vi "Scripting_ConnecorPaneRewiring.vi"(0 "ViRef":refnum<vi>, 1 "SubViThatHasChangedConnectorPane":path, 2 "OldConnectorPaneIndex":u32[](array[numeric]), 3 "NewConnectorPaneIndex":u32[](array[numeric]), 5 "error in (no error)":errorcluster) -> (19 "error out":errorcluster)   [LabVIEW 2020]
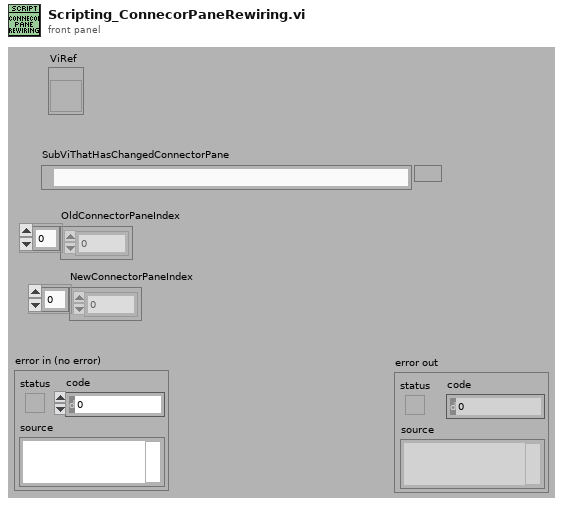
[diagram p1: front panel]
types:
  T1 = cluster{"New":refnum<vi>[], "Terminals[]":cluster{"Terminals[]":refnum<vi>[]}[]}
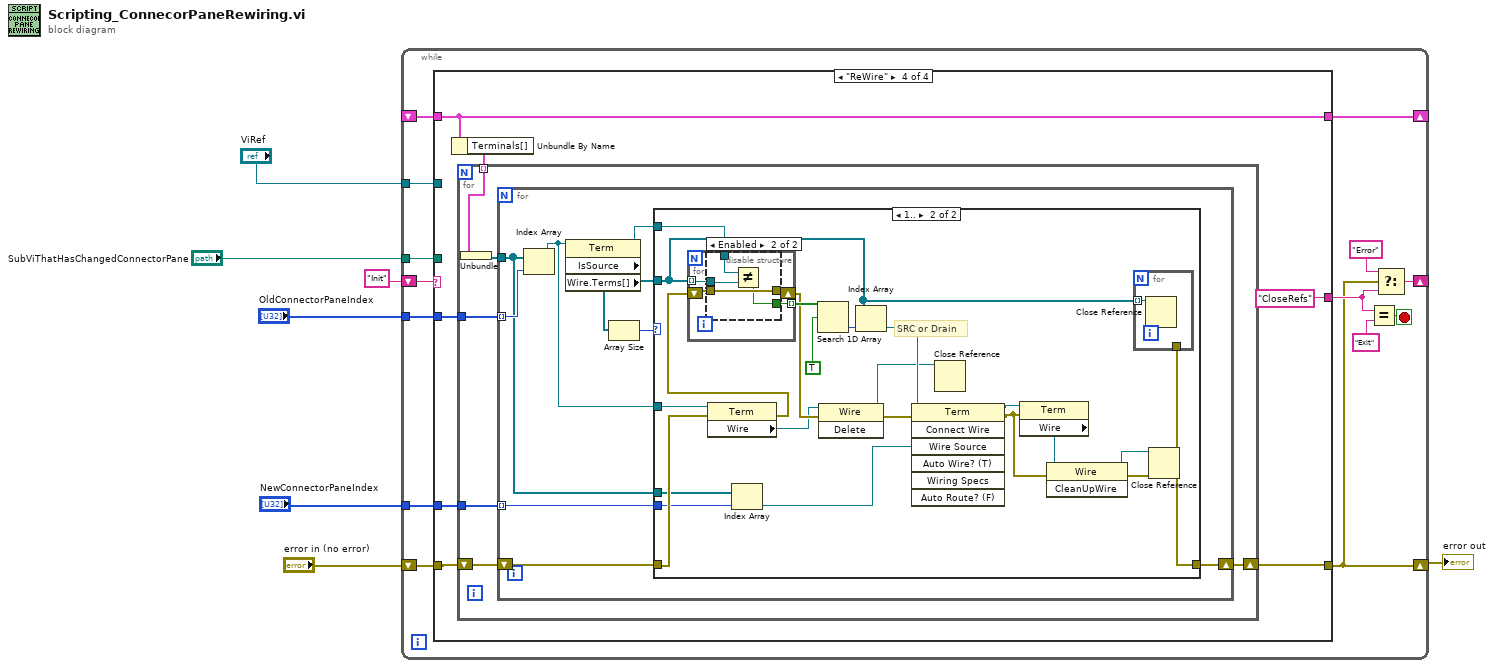
[diagram p0: block diagram]
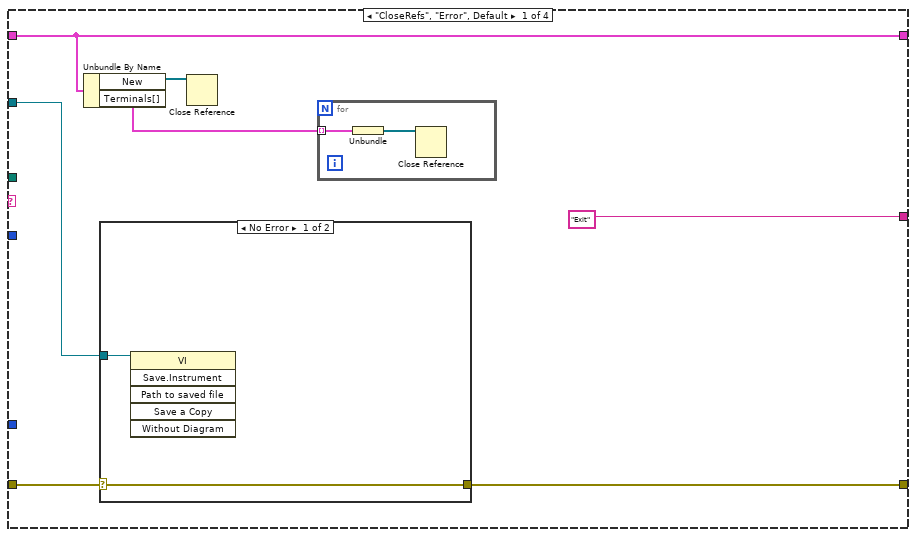
[diagram p2: hidden frame]
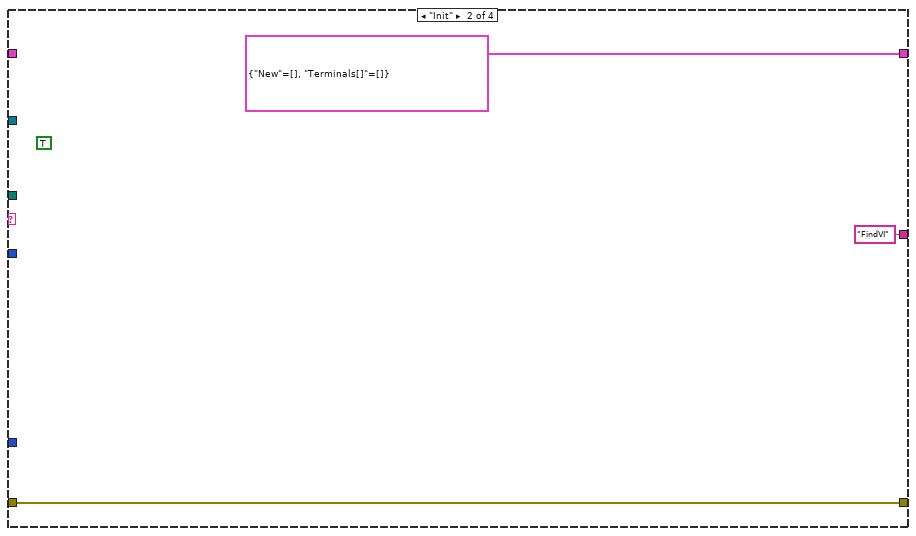
[diagram p4: hidden frame]
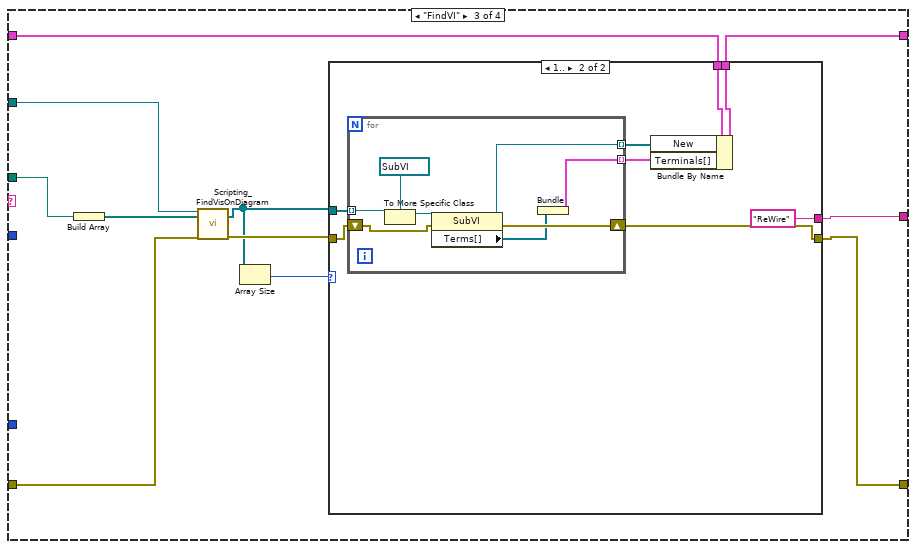
[diagram p5: hidden frame]
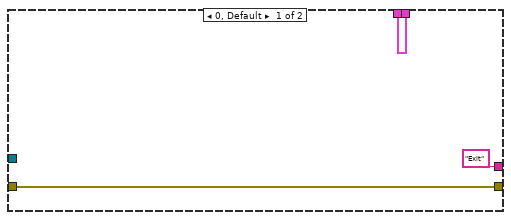
[diagram p6: hidden frame]
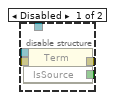
[diagram p8: hidden frame]
diagram:
  n1 = while {
    shift-right: [w14] -> w5
    shift-left: "error in (no error)" -> [w21]
    shift-right: [w19] -> _
    shift-left: "Init" -> [w20]
    shift-right: [w13] -> _
    shift-left: _ -> [w12]
    tunnel: "ViRef" -> [w11]
    tunnel: "SubViThatHasChangedConnectorPane" -> [w10]
    tunnel: "OldConnectorPaneIndex" -> [w9]
    tunnel: "NewConnectorPaneIndex" -> [w8]
    stop <- w18 stop-if-true
    n2 = case shown="\"ReWire\"" w20 {
      tunnel: w21 -> [w26 w35 w46 w69]
      tunnel: [w25 w35 w38 w68] -> w14
      tunnel: ["Exit" "FindVI" w37 "CloseRefs"] -> w15
      tunnel: [w27 T1 {"New"=[], "Terminals[]"=[]} w41 w73] -> w13
      tunnel: w12 -> [w27 _ w42 w73]
      tunnel: w11 -> [w24 _ w45 _]
      tunnel: w10 -> [_ _ w44 _]
      tunnel: w9 -> [_ _ _ w70]
      tunnel: w8 -> [_ _ _ w67]
      frame "CloseRefs", "Error", Default {
        n3 = Unbundle By Name(w27) -> ("New"=w22:refnum<vi>[], "Terminals[]"=w23:cluster{"Terminals[]":refnum<vi>[]}[])
        n4 = case shown="No Error" w26 {
          selector: w26 -> [w31 w33]
          tunnel: [w31 w33] -> w25
          tunnel: w24 -> [w32 _]
          frame No Error {
            n5 = invoke class="VI" method="Save.Instrument"(reference=w32) -> ()  [unwired: 5 in, 6 out]
          }
          frame Error {
          }
        }
        n6 = Close Reference(reference=w22) -> ()  [unwired: 1 in, 1 out]
        n7 = for {
          tunnel: w23 -> [w30] mode=indexing
          n8 = Unbundle(w30) -> ("Terminals[]"=w29:refnum<vi>[])
          n9 = Close Reference(reference=w29) -> ()  [unwired: 1 in, 1 out]
        }
      }
      frame "Init" {
        (unwired) TRUE ("Execution:Is Reentrant")
      }
      frame "FindVI" {
        n10 = Build Array(w44) -> (w43:path[])
        n11 = call <resource>:"Scripting_FindVisOnDiagram.vi"("ViRef"=w45, "VIsToSerachFor/ViName"=w43, "error in (no error)"=w46) -> ("VisFound"=w40:refnum<vi>[], "error out"=w47:errorcluster)  [unwired: 15 out]
        n12 = Array Size(array=w40) -> (size(s)=w39:i32)
        n13 = case shown="1.." w39 {
          tunnel: w47 -> [w49 w58]
          tunnel: w42 -> [w50 w57]
          tunnel: [w50 w56] -> w41
          tunnel: w40 -> [_ w55]
          tunnel: [w49 w54] -> w38
          tunnel: ["Exit" "ReWire"] -> w37
          frame 0, Default {
          }
          frame 1.. {
            n14 = for {
              tunnel: w55 -> [w61] mode=indexing
              tunnel: [w62] -> w53 mode=indexing
              tunnel: [w60] -> w52 mode=indexing
              shift-right: [w63] -> w54
              shift-left: w58 -> [w65]
              n15 = To More Specific Class(target class=refnum<vi> refnum ("WhileLoop"), reference=w61) -> (specific class reference=w66:refnum<vi>)  [unwired: 1 in, 1 out]
              n16 = property class="SubVI"(reference=w66, error in=w65) -> (reference out=w62:refnum<vi>, error out=w63:errorcluster, "Terms[]"=w59:refnum<vi>[])
              n17 = Bundle("Terms[]"=w59) -> (w60:cluster{"Terms[]":refnum<vi>[]})  [unwired: 1 in]
            }
            n18 = Bundle By Name(cluster=w57, "New"=w53, "Terminals[]"=w52) -> (w56:T1)
          }
        }
      }
      frame "ReWire" {
        n19 = Unbundle By Name(w73) -> ("Terminals[]"=w71:cluster{"Terminals[]":refnum<vi>[]}[])
        n20 = for {
          tunnel: w71 -> [w79] mode=indexing
          tunnel: w70 -> [w78]
          tunnel: w67 -> [w75]
          shift-right: [w76] -> w68
          shift-left: w69 -> [w77]
          n21 = Unbundle(w79) -> ("Terminals[]"=w74:refnum<vi>[])
          n22 = for {
            tunnel: w74 -> [w83]
            tunnel: w78 -> [w88] mode=indexing
            shift-right: [w85] -> w76
            shift-left: w77 -> [w86]
            tunnel: w75 -> [w82] mode=indexing
            n23 = Index Array(array=w83, index=w88) -> (element=w81:refnum<vi>)
            n24 = property class="Term" props=["IsSource", "Wire", "Terms[]"](reference=w81) -> (reference out=w80:refnum<vi>, "Wire.Terms[]"=w84:refnum<vi>[])  [unwired: 1 in, 2 out]
            n25 = Array Size(array=w84) -> (size(s)=w87:i32)
            n26 = case shown="1.." w87 {
              tunnel: w86 -> [w89 w107]
              tunnel: [w89 w92] -> w85
              tunnel: w84 -> [_ w98]
              tunnel: w81 -> [_ w109]
              tunnel: w83 -> [_ w106]
              tunnel: w82 -> [_ w105]
              tunnel: w80 -> [_ w90]
              frame 0, Default {
              }
              frame 1.. {
                # "SRC or Drain"
                n27 = property class="Term"(reference=w109, error in=w107) -> (error out=w108:errorcluster, "Wire"=w100:refnum<vi>)  [unwired: 1 out]
                n28 = for {
                  tunnel: w98 -> [w117] mode=indexing
                  tunnel: [w116] -> w111 mode=indexing
                  shift-right: [w114] -> w104
                  shift-left: w108 -> [w115]
                  tunnel: w90 -> [w113]
                  n29 = disable-structure shown="Enabled" {
                    disable-tunnel: w117 -> [w121 w124]
                    disable-tunnel: [w120 w122] -> w116
                    disable-tunnel: w115 -> [w119 w125]
                    disable-tunnel: [w118 w125] -> w114
                    disable-tunnel: w113 -> [_ w123]
                    frame Disabled {
                      n30 = property class="Term"(reference=w121, error in=w119) -> (error out=w118:errorcluster, "IsSource"=w120:bool)  [unwired: 1 out]
                    }
                    frame Enabled {
                      n31 = Not Equal?(x=w123, y=w124) -> (x != y?=w122:bool)
                    }
                  }
                }
                n32 = Index Array(array=w106, index=w105) -> (element=w101:refnum<vi>)
                n33 = Search 1D Array(1D array=w111, element=TRUE) -> (index of element=w110:i32)  [unwired: 1 out]
                n34 = invoke class="Wire" method="Delete"(reference=w100, error in=w104) -> (reference out=w99:refnum<vi>, error out=w103:errorcluster)  [unwired: 1 in, 1 out]
                n35 = Index Array(array=w98, index=w110) -> (element=w102:refnum<vi>)
                n36 = invoke class="Term" method="Connect Wire"(reference=w102, error in=w103, "Wire Source"=w101) -> (reference out=w97:refnum<vi>, error out=w93:errorcluster)  [unwired: 4 in, 5 out]
                n37 = Close Reference(reference=w99) -> ()  [unwired: 1 in, 1 out]
                n38 = property class="Term"(reference=w97, error in=w93) -> ("Wire"=w96:refnum<vi>)  [unwired: 2 out]
                n39 = invoke class="Wire" method="CleanUpWire"(reference=w96, error in=w93) -> (reference out=w94:refnum<vi>, error out=w95:errorcluster)  [unwired: 1 in, 1 out]
                n40 = Close Reference(reference=w94, error in (no error)=w95) -> (error out=w92:errorcluster)
                n41 = for {
                  tunnel: w92 -> [_]
                  tunnel: w98 -> [w112] mode=indexing
                  n42 = Close Reference(reference=w112) -> ()  [unwired: 1 in, 1 out]
                }
              }
            }
          }
        }
      }
    }
    n43 = Equal?(x=w15, y="Exit") -> (x = y?=w18:bool)
    n44 = Select(t="Error", s=w14, f=w15) -> (s? t:f=w19:string)
  }
  "error out" <- w5
